vi "Update System Errors Indicator.vi"(8 "error in (no error)":errorcluster, 10 "System Errors":bool, 11 "CIF_UI in":refnum<class "CIF_Manager_UI.lvclass">) -> (0 "error out":errorcluster)   [LabVIEW 2021, in "CIF_Manager_UI.lvclass"]
uses:
  CIF_Manager_UI.lvclass
  CIF_Manager_UI.lvclass/CIF_Manager_UI.ctl
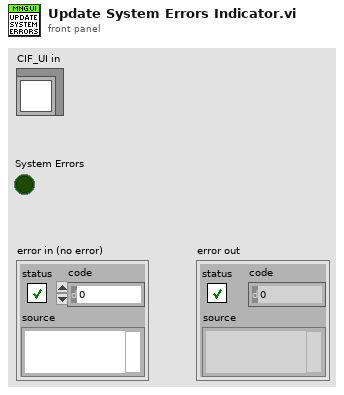
[diagram p1: front panel]
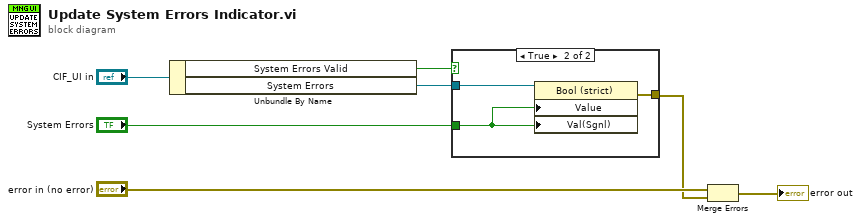
[diagram p0: block diagram]
diagram:
  n1 = Unbundle By Name("CIF_UI in") -> ("System Errors Valid"=w5:bool, "System Errors"=w4:refnum<vi>)
  n2 = case shown="True" w5 {
    tunnel: w4 -> [_ w10]
    tunnel: "System Errors" -> [_ w9]
    tunnel: [_ w8] -> w2
    frame False {
    }
    frame True {
      n3 = property class="Bool (strict)"(reference=w10, "Value"=w9, "Val(Sgnl)"=w9) -> (error out=w8:errorcluster)  [unwired: 1 in, 1 out]
    }
  }
  n4 = Merge Errors("error in (no error)", w2) -> (→"error out":errorcluster)
